vi "Pre Launch Init.vi"(11 "CCD Configuration in":refnum<class "CCD Configuration.lvclass">) -> (0 "error out":errorcluster, 3 "CCD Configuration out":refnum<class "CCD Configuration.lvclass">)   [LabVIEW 2016, in "Hardware.lvlib" / "CCD.lvlib" / "CCD Configuration.lvclass"]
doc: "(<B>Filename</B>: Actor Framework.lvlib:Actor.lvclass:Pre Launch Init.vi)\n\nDefines behavior that occurs after the Launch Nested Actor method is invoked but before the actor's Actor Core method begins running.\n\nBy default, this method does nothing. A descendant class may override it to define behavior."
uses:
  <userlib>/Common Components/Hardware/CCD/CCD Configuration.lvclass
  <userlib>/Configuration Dialog Actor/Configuration.lvclass
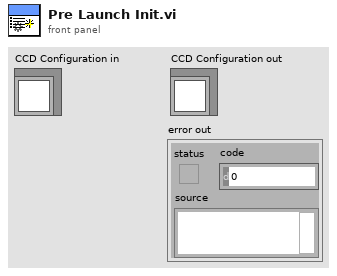
[diagram p1: front panel]
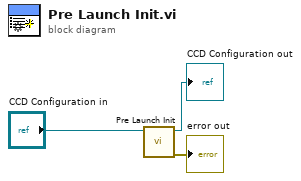
[diagram p0: block diagram]
diagram:
  n1 = call-parent "Pre Launch Init.vi"("Actor in"="CCD Configuration in") -> ("error out"=→"error out":errorcluster, "Actor out"=→"CCD Configuration out":refnum<class "CCD Configuration.lvclass">)  [unwired: 9 in]
